vi "Image display gain-offset - SubVI.vi"(0 "Image In":T1, 1 "Autoscale?":bool, 2 "Display Type (s)":enum16{"Front Panel", "Separate Window"}(ring), 3 "Mode":enum16{"Setup", "Run"}(ring), 5 "Black/White Levels Ctl Ref (s)":refnum<vi>, 6 "Zoom +":bool, 7 "Auto Resize to Image Size?\n(Window only)":bool=TRUE, 8 "Zoom -":bool, 10 "Auto position\n(Window only)":bool=TRUE, 11 "error in (s)":errorcluster, 12 "Pixel depth (s)":u32, 13 "Window Title\n(Window only)":string, 14 "Window Number\n(Window only)":i32) -> (4 "Image Out":T1, 15 "error out":errorcluster)   [LabVIEW 2014]
doc: "Initializes and displays images (8- or 16-bit monochrome) in a front panel image indicator or a separate window. Gain and offset of the image are set by a Black/White level slider on the caller's front panel, a ref to which is passed to this vi.\n\nIntended for non-interactive use only. Can be used in plug-ins."
uses:
  <vilib>/vision/Image Controls.llb/IMAQ Image.ctl
panel:
  in  "Image Control Ref\n(Panel Only)":refnum<vi>
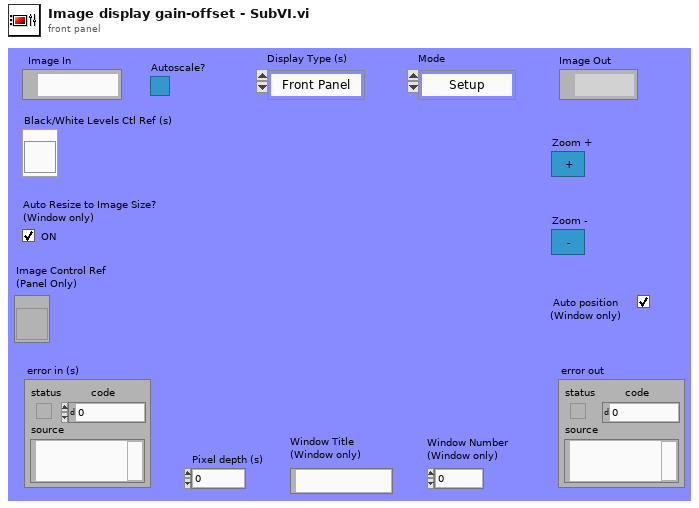
[diagram p1: front panel]
types:
  T1 = typedef "IMAQ Image.ctl" = refnum<image>
  T2 = enum32{"No Selection", "Point", "Line", "Rectangle", "Oval", "Polygon", "Free", "Unused1", "Zoom", "Unused2", "Broken Line", "Free Hand Line"}
  T3 = cluster{"Conversion Method":u32, "Minimum Value":i32, "Maximum Value":i32, "# Shifts":i32}
  T4 = enum32{"No Selection", "Point", "Line", "Rectangle", "Oval", "Polygon", "Free", "Unused1", "Zoom", "Unused2", "Broken Line", "Free Hand Line"}[]
  T5 = typedef "LVRectTypeDef.ctl" = cluster{"Left":i16, "Top":i16, "Right":i16, "Bottom":i16}
  T6 = cluster{"Mean Value":sgl, "Standard Variation":sgl, "Minimal Value":sgl, "Maximal Value":sgl, "Area (calibrated)":sgl, "Area (pixels)":i32, "%":sgl}
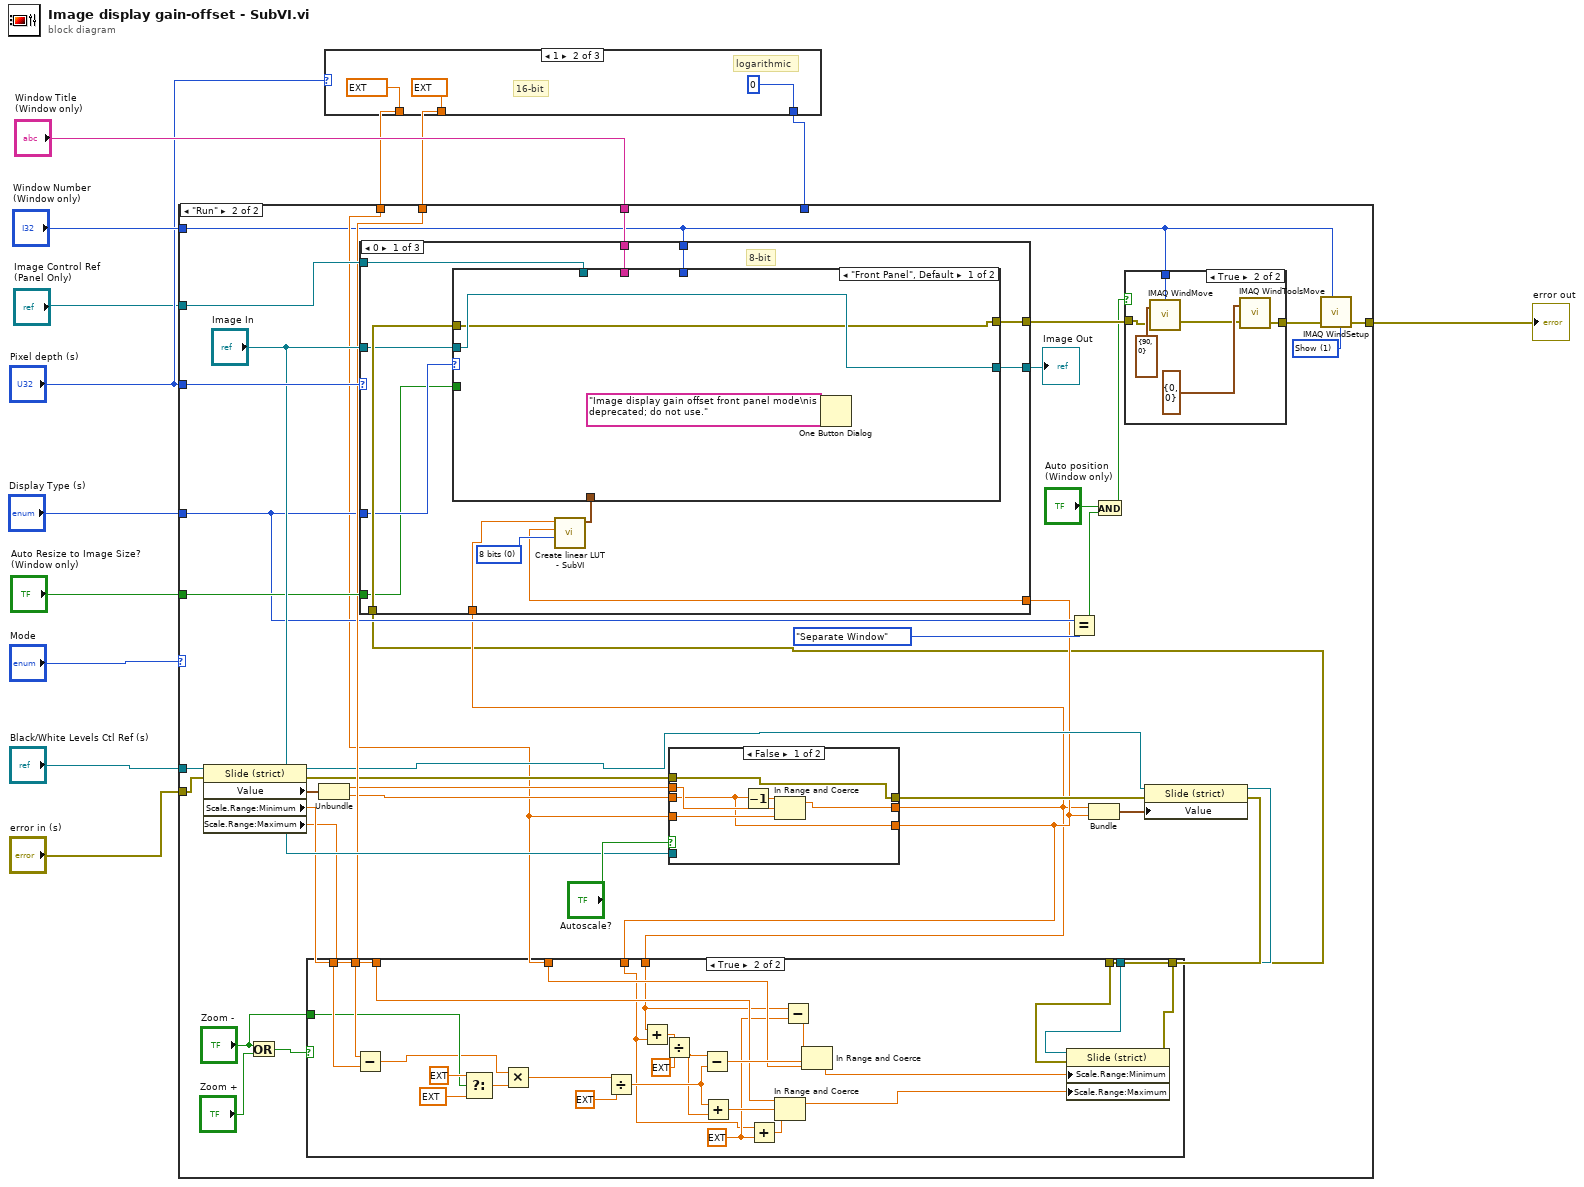
[diagram p0: block diagram]
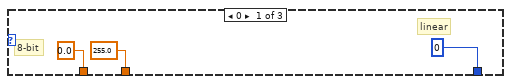
[diagram p2: hidden frame]
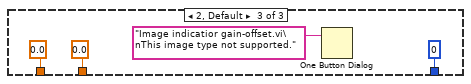
[diagram p3: hidden frame]
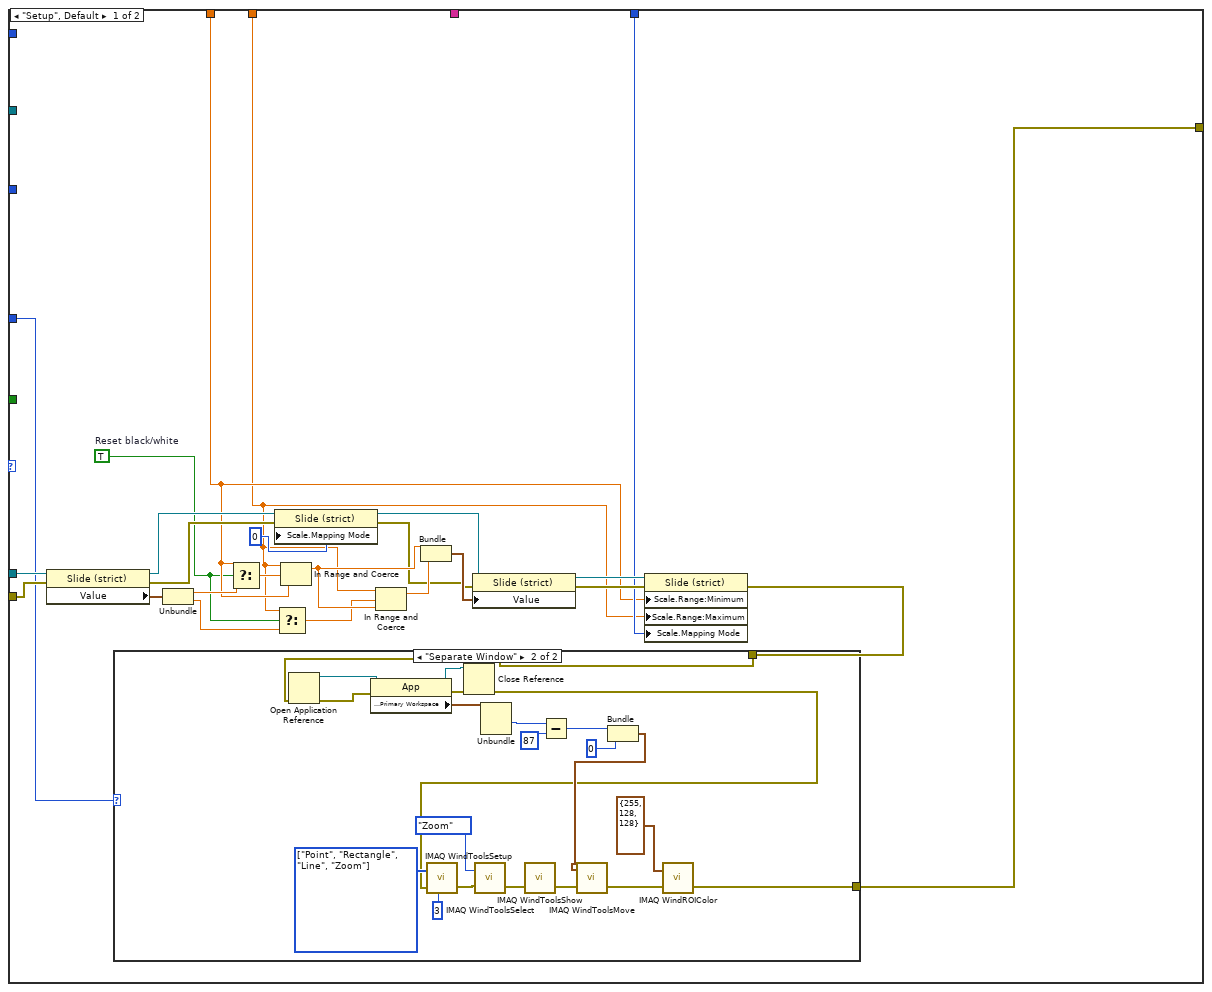
[diagram p4: hidden frame]
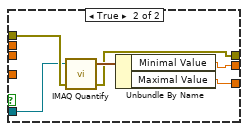
[diagram p8: hidden frame]
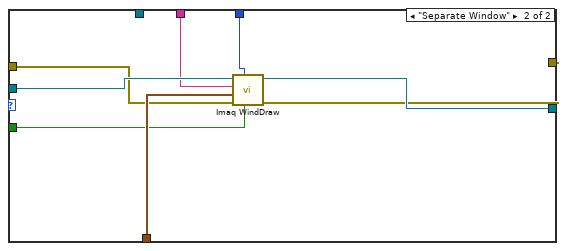
[diagram p9: hidden frame]
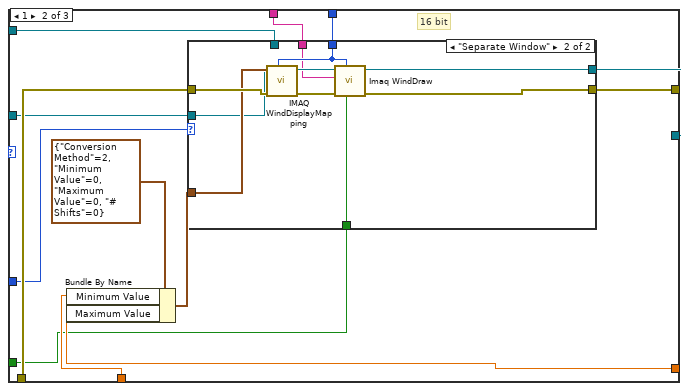
[diagram p10: hidden frame]
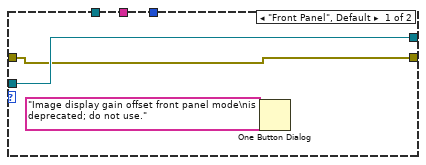
[diagram p11: hidden frame]
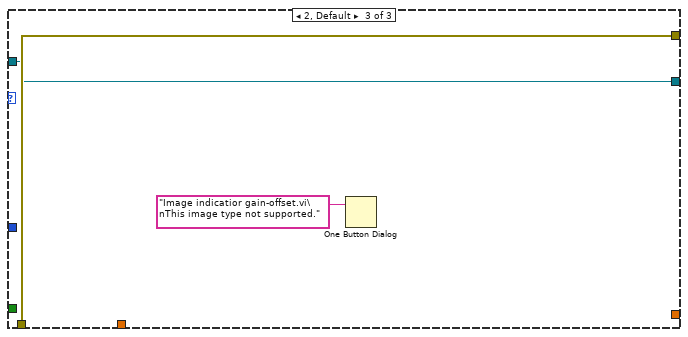
[diagram p12: hidden frame]
diagram:
  n1 = case shown="1" "Pixel depth (s)" {
    tunnel: [0.0 ("lower limit") ext -32768.0 ("lower limit") 0.0 ("lower limit")] -> w4
    tunnel: [255.0 ("lower limit") ext 32767.0 ("lower limit") 0.0 ("lower limit")] -> w3
    tunnel: [u8 0 ("Scale.Mapping Mode") u8 0 ("Scale.Mapping Mode") u8 0 ("Scale.Mapping Mode")] -> w2
    frame 0 {
      # "linear"
      # "8-bit"
    }
    frame 1 {
      # "16-bit"
      # "logarithmic"
    }
    frame 2, Default {
      n2 = One Button Dialog(message="Image indicatior gain-offset.vi\nThis image type not supported.") -> ()  [unwired: 2 out]
    }
  }
  n3 = case shown="\"Run\"" "Mode" {
    tunnel: [w33 w88] -> w13
    tunnel: "Pixel depth (s)" -> [_ w106]
    tunnel: "Image Control Ref\n(Panel Only)" -> [_ w105]
    tunnel: "Black/White Levels Ctl Ref (s)" -> [w47 w104]
    tunnel: "error in (s)" -> [w46 w103]
    tunnel: "Display Type (s)" -> [w32 w84]
    tunnel: "Window Number\n(Window only)" -> [_ w70]
    tunnel: "Auto Resize to Image Size?\n(Window only)" -> [_ w98]
    tunnel: "Window Title\n(Window only)" -> [_ w97]
    tunnel: w4 -> [w28 w72]
    tunnel: w3 -> [w25 w91]
    tunnel: w2 -> [w35 _]
    frame "Setup", Default {
      w24 = TRUE  # Reset black/white
      n4 = property class="Slide (strict)"(reference=w47, error in=w46) -> (reference out=w39:refnum<vi>, error out=w38:errorcluster, "Value"=w45:cluster{ext, ext})
      n5 = Unbundle(w45) -> (w29:ext, w27:ext)
      n6 = Select(t=w28, s=w24, f=w29) -> (s? t:f=w30:ext)
      n7 = property class="Slide (strict)"(reference=w39, error in=w38, "Scale.Mapping Mode"=u8 0) -> (reference out=w36:refnum<vi>, error out=w37:errorcluster)
      n8 = Select(t=w25, s=w24, f=w27) -> (s? t:f=w26:ext)
      n9 = In Range and Coerce(upper limit=w25, x=w30, lower limit=w28) -> (coerced(x)=w42:ext)  [unwired: 1 out]
      n10 = In Range and Coerce(upper limit=w25, x=w26, lower limit=w42) -> (coerced(x)=w41:ext)  [unwired: 1 out]
      n11 = Bundle("lower limit"=w42, "lower limit"=w41) -> (w40:cluster{"lower limit":ext, "lower limit":ext})  [unwired: 1 out]
      n12 = property class="Slide (strict)"(reference=w36, error in=w37, "Value"=w40) -> (reference out=w44:refnum<vi>, error out=w43:errorcluster)
      n13 = property class="Slide (strict)"(reference=w44, error in=w43, "Scale.Range:Minimum"=w28, "Scale.Range:Maximum"=w25, "Scale.Mapping Mode"=w35) -> (error out=w34:errorcluster)  [unwired: 1 out]
      n14 = case shown="\"Separate Window\"" w32 {
        tunnel: w34 -> [w48 w50]
        tunnel: [w48 w49] -> w33
        frame "Front Panel", Default {
        }
        frame "Separate Window" {
          w63 = T4 [enum."Point", enum."Rectangle", enum."Line", enum."Zoom"] items=["No Selection", "Point", "Line", "Rectangle", "Oval", "Polygon", "Free", "Unused1", "Zoom", "Unused2", "Broken Line", "Free Hand Line"] ("Tools")
          n15 = Open Application Reference(8:w50) -> (0:w58:errorcluster, 3:w61:refnum<vi>)  [unwired: 3 out]
          n16 = property class="App"(reference=w61, error in=w58) -> (reference out=w57:refnum<vi>, error out=w59:errorcluster, "Display:Primary Workspace"=w60:T5)
          n17 = Close Reference(reference=w57, error in (no error)=w59) -> (error out=w51:errorcluster)
          n18 = call "IMAQ WindToolsSetup"("Tools"=w63, "Icons per Line (4)"=3, "error in (no error)"=w51) -> ("error out"=w64:errorcluster)  [unwired: 1 in, 2 out]
          n19 = call "IMAQ WindToolsSelect"("Tool (Point)"=T2."Zoom", "error in (no error)"=w64) -> ("error out"=w65:errorcluster)  [unwired: 2 in, 2 out]
          n20 = Unbundle(w60) -> ("Right"=w56:i16)  [unwired: 3 out]
          n21 = call "IMAQ WindToolsShow"("error in (no error)"=w65) -> ("error out"=w67:errorcluster)  [unwired: 2 in, 3 out]
          n22 = Subtract(x=w56, y=i16 87) -> (x-y=w54:i16)
          n23 = Bundle(w54, "X Position"=0) -> (w52:cluster{i16, "X Position":i32})  [unwired: 1 out]
          n24 = call "IMAQ WindToolsMove"("Coordinates"=w52, "error in (no error)"=w67) -> ("error out"=w62:errorcluster)  [unwired: 1 in, 3 out]
          n25 = call "IMAQ WindROIColor"("Color of ROI (white)"=cluster{"Red":u8, "Green":u8, "Blue":u8} {"Red"=255, "Green"=128, "Blue"=128}, "error in (no error)"=w62) -> ("error out"=w49:errorcluster)  [unwired: 4 out]
        }
      }
    }
    frame "Run" {
      w71 = 1 items=["Hide", "Show", "No change"] ("Scrollbars (No change)")
      n26 = property class="Slide (strict)"(reference=w104, error in=w103) -> (reference out=w79:refnum<vi>, error out=w80:errorcluster, "Value"=w102:cluster{ext, ext}, "Scale.Range:Minimum"=w96:dbl, "Scale.Range:Maximum"=w95:dbl)
      n27 = Or(x="Zoom -", y="Zoom +") -> (x .or. y?=w94:bool)
      n28 = Unbundle(w102) -> (w77:ext, w90:ext)
      n29 = case shown="False" "Autoscale?" {
        tunnel: w80 -> [w142 w152]
        tunnel: "Image In" -> [_ w151]
        tunnel: w77 -> [w145 _]
        tunnel: w90 -> [w143 _]
        tunnel: w72 -> [w146 _]
        tunnel: [w144 w150] -> w76
        tunnel: [w143 w149] -> w78
        tunnel: [w142 w148] -> w81
        frame False {
          n30 = Decrement(x=w143) -> (x-1=w147:ext)
          n31 = In Range and Coerce(upper limit=w147, x=w145, lower limit=w146) -> (coerced(x)=w144:ext)  [unwired: 1 out]
        }
        frame True {
          n32 = call "IMAQ Quantify"("error in (no error)"=w152, "Image"=w151) -> ("error out"=w148:errorcluster, "Global Report"=w153:T6)  [unwired: 1 in, 1 out]
          n33 = Unbundle By Name(w153) -> ("Minimal Value"=w150:sgl, "Maximal Value"=w149:sgl)
        }
      }
      n34 = Equal?(x=w84, y=enum16{"Front Panel", "Separate Window"}."Separate Window") -> (x = y?=w85:bool)
      n35 = Bundle("lower limit"=w76, "Maximal Value"=w78) -> (w82:cluster{"lower limit":ext, "Maximal Value":ext})  [unwired: 1 out]
      n36 = And(x="Auto position\n(Window only)", y=w85) -> (x .and. y?=w87:bool)
      n37 = property class="Slide (strict)"(reference=w79, error in=w81, "Value"=w82) -> (reference out=w74:refnum<vi>, error out=w75:errorcluster)
      n38 = case shown="True" w94 {
        tunnel: w96 -> [_ w139]
        tunnel: w95 -> [_ w138]
        tunnel: "Zoom -" -> [_ w135]
        tunnel: w91 -> [_ w122]
        tunnel: w76 -> [_ w116]
        tunnel: w78 -> [_ w117]
        tunnel: w75 -> [w114 w127]
        tunnel: w74 -> [_ w126]
        tunnel: [w114 w125] -> w73
        tunnel: w72 -> [_ w121]
        frame False {
        }
        frame True {
          w118 = ext 20.0 ("y")
          n39 = Subtract(x=w138, y=w139) -> (x-y=w133:dbl)
          n40 = Select(t=ext 4.0, s=w135, f=ext 0.25) -> (s? t:f=w134:ext)
          n41 = Multiply(x=w133, y=w134) -> (x*y=w115:ext)
          n42 = Divide(x=w115, y=ext 2.0) -> (x/y=w131:ext)
          n43 = Add(x=w116, y=w117) -> (x+y=w141:ext)
          n44 = Divide(x=w141, y=ext 2.0) -> (x/y=w130:ext)
          n45 = Subtract(x=w130, y=w131) -> (x-y=w128:ext)
          n46 = Add(x=w131, y=w130) -> (x+y=w129:ext)
          n47 = Add(x=w117, y=w118) -> (x+y=w120:ext)
          n48 = In Range and Coerce(upper limit=w122, x=w129, lower limit=w120) -> (coerced(x)=w124:ext)  [unwired: 1 out]
          n49 = Subtract(x=w116, y=w118) -> (x-y=w119:ext)
          n50 = In Range and Coerce(upper limit=w119, x=w128, lower limit=w121) -> (coerced(x)=w123:ext)  [unwired: 1 out]
          n51 = property class="Slide (strict)"(reference=w126, error in=w127, "Scale.Range:Minimum"=w123, "Scale.Range:Maximum"=w124) -> (error out=w125:errorcluster)  [unwired: 1 out]
        }
      }
      n52 = case shown="0" w106 {
        tunnel: [w166 w186 w204] -> w89
        tunnel: w105 -> [w164 w189 _]
        tunnel: w73 -> [w163 w187 w204]
        tunnel: w84 -> [w161 w185 _]
        tunnel: "Image In" -> [w160 w183 w203]
        tunnel: [w159 w181 w203] -> w99
        tunnel: w70 -> [w158 w184 _]
        tunnel: w98 -> [w157 w178 _]
        tunnel: w97 -> [w156 w182 _]
        tunnel: w78 -> [w155 w179 _]
        tunnel: w76 -> [w154 w180 _]
        frame 0 {
          w162 = u32 0 items=["8 bits", "16 bits", "Float", "Complex", "RGB", "HSL"] ("Image Type")
          # "8-bit"
          n53 = call "Create linear LUT - SubVI.vi"("Input Image Type"=w162, "White Value"=w155, "Black Value"=w154) -> ("Palette Out"=w165:cluster{"Red":u8, "Green":u8, "Blue":u8}[])  [unwired: 5 in, 1 out]
          n54 = case shown="\"Front Panel\", Default" w161 {
            tunnel: [w167 w170] -> w166
            tunnel: w165 -> [_ w177]
            tunnel: w164 -> [_ _]
            tunnel: w163 -> [w167 w171]
            tunnel: w160 -> [w169 w176]
            tunnel: [w169 w175] -> w159
            tunnel: w158 -> [_ w174]
            tunnel: w157 -> [_ w173]
            tunnel: w156 -> [_ w172]
            frame "Front Panel", Default {
              n55 = One Button Dialog(message="Image display gain offset front panel mode\nis deprecated; do not use.") -> ()  [unwired: 1 in, 1 out]
            }
            frame "Separate Window" {
              n56 = call "Imaq WindDraw"("Resize to Image Size? (Y)"=w173, "Window Number (0...15)"=w174, "error in (no error)"=w171, "Color Palette"=w177, "Title"=w172, "Image"=w176) -> ("error out"=w170:errorcluster, "Image Out (duplicate)"=w175:T1)  [unwired: 4 out]
            }
          }
        }
        frame 1 {
          # "16 bit"
          n57 = Bundle By Name(cluster=T3 {"Conversion Method"=2, "Minimum Value"=0, "Maximum Value"=0, "# Shifts"=0} ("Conversion Policy (Full Dynamic)"), "Minimum Value"=w180, "Maximum Value"=w179) -> (w188:T3)
          n58 = case shown="\"Separate Window\"" w185 {
            tunnel: w189 -> [_ _]
            tunnel: w188 -> [_ w199]
            tunnel: w187 -> [w192 w201]
            tunnel: [w192 w200] -> w186
            tunnel: w184 -> [_ w198]
            tunnel: w183 -> [w193 w197]
            tunnel: w182 -> [_ w196]
            tunnel: [w193 w195] -> w181
            tunnel: w178 -> [_ w194]
            frame "Front Panel", Default {
              n59 = One Button Dialog(message="Image display gain offset front panel mode\nis deprecated; do not use.") -> ()  [unwired: 1 in, 1 out]
            }
            frame "Separate Window" {
              n60 = call "IMAQ WindDisplayMapping"("Window Number (0...15)"=w198, "error in (no error)"=w201, "Conversion Policy (Default)"=w199) -> ("error out"=w202:errorcluster)  [unwired: 1 in, 7 out]
              n61 = call "Imaq WindDraw"("Resize to Image Size? (Y)"=w194, "Window Number (0...15)"=w198, "error in (no error)"=w202, "Title"=w196, "Image"=w197) -> ("error out"=w200:errorcluster, "Image Out (duplicate)"=w195:T1)  [unwired: 1 in, 4 out]
            }
          }
        }
        frame 2, Default {
          n62 = One Button Dialog(message="Image indicatior gain-offset.vi\nThis image type not supported.") -> ()  [unwired: 2 out]
        }
      }
      "Image Out" <- w99
      n63 = case shown="True" w87 {
        tunnel: w89 -> [w107 w112]
        tunnel: [w107 w110] -> w88
        tunnel: w70 -> [_ w109]
        frame False {
        }
        frame True {
          n64 = call "IMAQ WindMove"("Window Number (0...15)"=w109, "Coordinates (screen)"=cluster{"X Position":i32, "Y Position":i32} {"X Position"=90, "Y Position"=0}, "error in (no error)"=w112) -> ("error out"=w108:errorcluster)  [unwired: 1 in, 2 out]
          n65 = call "IMAQ WindToolsMove"("Coordinates"=cluster{"X Position":i32, "Y Position":i32} {"X Position"=0, "Y Position"=0}, "error in (no error)"=w108) -> ("error out"=w110:errorcluster)  [unwired: 1 in, 3 out]
        }
      }
      n66 = call "IMAQ WindSetup"("Scrollbars (No change)"=w71, "Window Number (0...15)"=w70) -> ()  [unwired: 5 in, 5 out]
    }
  }
  "error out" <- w13
